vi "Unload.vi"(8 "error in (no error)":errorcluster, 10 "Unload":string, 11 "Sequencing in":refnum<class "Sequencing.lvclass">) -> (0 "error out":errorcluster, 3 "Sequencing out":refnum<class "Sequencing.lvclass">)   [LabVIEW 2020, in "VolatusSeq.lvlib" / "Sequencing.lvclass"]
uses:
  Sequencing.lvclass
  Sequencing.lvclass/Sequencing.ctl
  Sequence/Sequence.lvclass
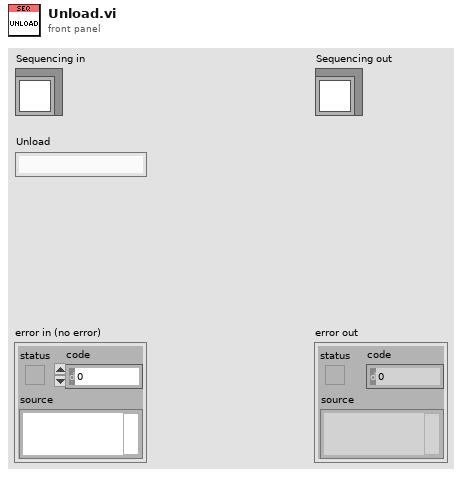
[diagram p1: front panel]
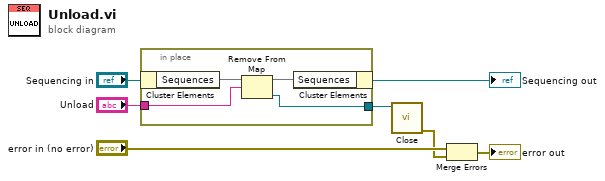
[diagram p0: block diagram]
diagram:
  n1 = in-place {
    in-place-border: "Unload" -> [w10]
    in-place-border: [w8] -> w4
    n2 = in-place-cluster #1("Sequencing in") -> ("Sequences"=w11:map{string, refnum<class "Sequence.lvclass">})
    n3 = Remove From Map(10:w10, 11:w11) -> (1:w8:refnum<class "Sequence.lvclass">, 3:w9:map{string, refnum<class "Sequence.lvclass">})  [unwired: 1 out]
    n4 = in-place-cluster #1("Sequences"=w9) -> (→"Sequencing out":refnum<class "Sequencing.lvclass">)
  }
  n5 = call "Close.vi"("Sequence in"=w4) -> ("error out"=w1:errorcluster)  [unwired: 9 in, 1 out]
  n6 = Merge Errors("error in (no error)", w1) -> (→"error out":errorcluster)
